vi "WaveTank.vi"() -> ()   [LabVIEW 2025]
uses:
  install/bin/libwavetanktestinglib.dll
panel:
  in  "WT_InputFile":string="..\\..\\python\\wavetankconfig.in"
  out "ErrMsg":string="C:\\Users\\schamot\\Desktop\\openfast\\reg_tests\\r-test\\glue-codes\\openfast\\MHK_RM1_Floating\\MHK_RM1_Floating_MoorDyn.dat"
  out "path":path
  out "Application Directory":path
  out "ErrStat":i32
  in  "Testing in":errorcluster
  out "Testing Out":errorcluster
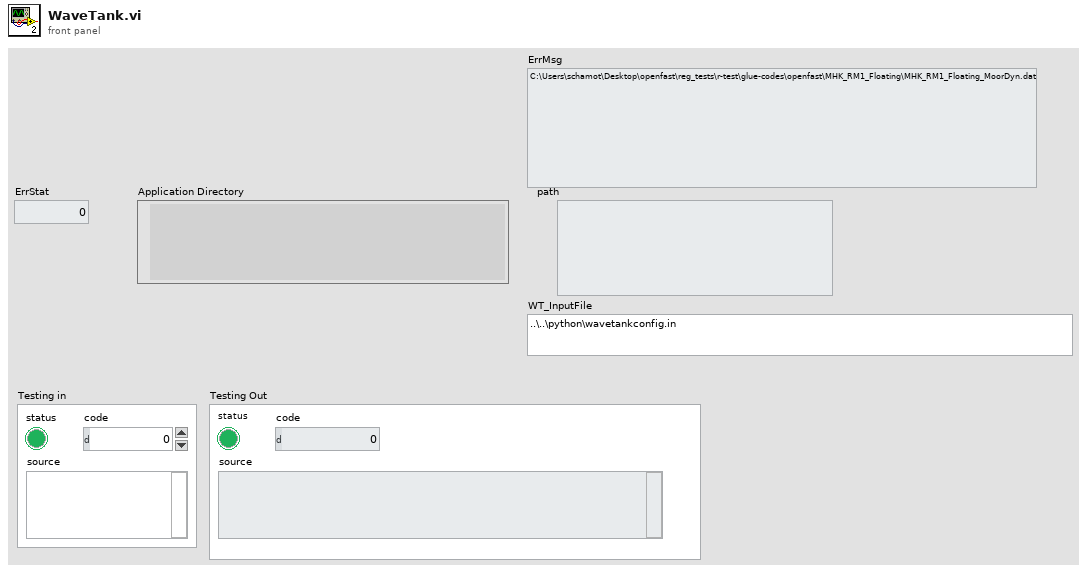
[diagram p1: front panel]
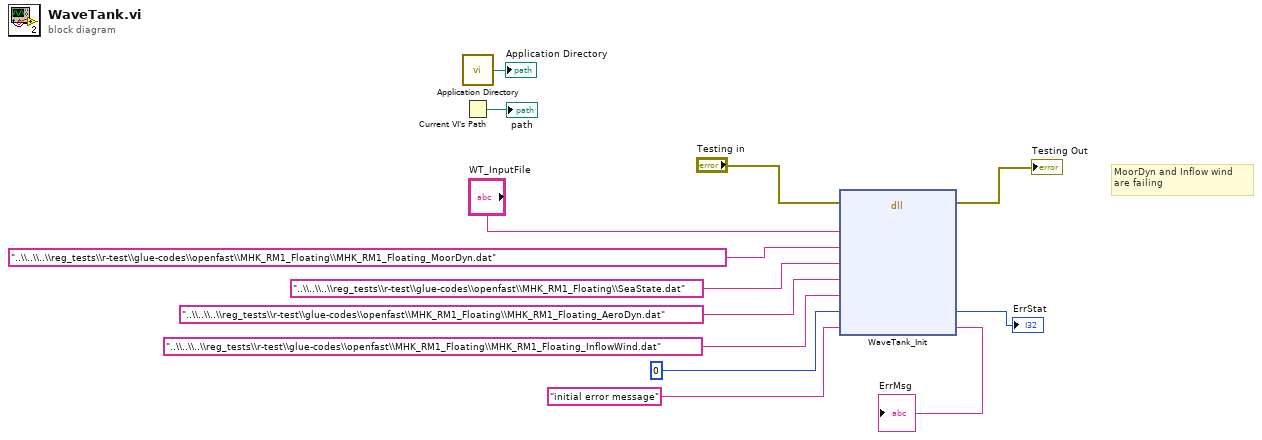
[diagram p0: block diagram]
diagram:
  # "MoorDyn and Inflow wind\nare failing"
  n1 = call <vilib>:"Application Directory.vi"() -> ("Application Directory"=→"Application Directory":path)
  n2 = Current VI's Path() -> (path=→"path":path)
  n3 = dll-call lib="C:/Users/aplatt/Documents/software-development/GitHub/openfast/install/bin/libwavetanktestinglib.dll" fn="WaveTank_Init"(error in="Testing in", "WT_InputFile_C"="WT_InputFile", "MD_InputFile_C"="..\\..\\..\\reg_tests\\r-test\\glue-codes\\openfast\\MHK_RM1_Floating\\MHK_RM1_Floating_MoorDyn.dat" ("MD"), "SS_InputFile_C"="..\\..\\..\\reg_tests\\r-test\\glue-codes\\openfast\\MHK_RM1_Floating\\SeaState.dat" ("SS"), "AD_InputFile_C"="..\\..\\..\\reg_tests\\r-test\\glue-codes\\openfast\\MHK_RM1_Floating\\MHK_RM1_Floating_AeroDyn.dat" ("AD"), "IfW_InputFile_C"="..\\..\\..\\reg_tests\\r-test\\glue-codes\\openfast\\MHK_RM1_Floating\\MHK_RM1_Floating_InflowWind.dat" ("IfW"), "ErrStat_C"=0, "ErrMsg_C"="initial error message") -> (error out=→"Testing Out":errorcluster, "ErrStat_C"=→"ErrStat":i32, "ErrMsg_C"=→"ErrMsg":string)  [unwired: 8 in, 1 out]
